vi "Instrucoes.vi"() -> ()   [LabVIEW 2011]
doc: "Esse VI mostra instruções do jogo."
panel:
  in  "OK":bool
  out "Instruções":string
  # "Instruções"
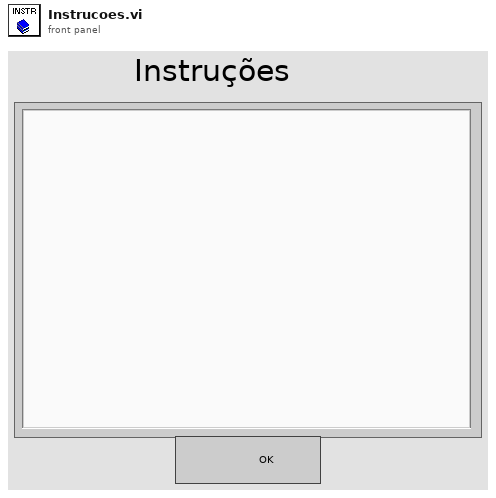
[diagram p1: front panel]
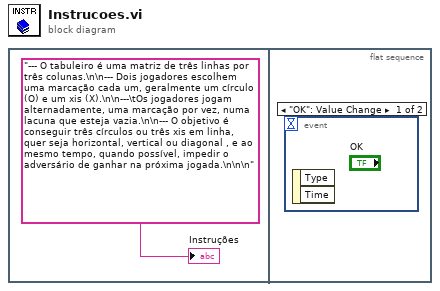
[diagram p0: block diagram]
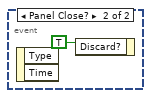
[diagram p2: hidden frame]
diagram:
  n1 = flat-sequence {
    frame #0 {
      "Instruções" <- "--- O tabuleiro é uma matriz de três linhas por três colunas.\n\n--- Dois jogadores escolhem uma marcação cada um, geralmente um círculo (O) e um xis (X).\n\n---\tOs jogadores jogam alternadamente, uma marcação por vez, numa lacuna que esteja vazia.\n\n--- O objetivo é conseguir três círculos ou três xis em linha, quer seja horizontal, vertical ou diagonal , e ao mesmo tempo, quando possível, impedir o adversário de ganhar na próxima jogada.\n\n\n" ("Instruções")
    }
    frame #1 {
      n2 = event shown="[0] \"OK\": Value Change" {
        selector: _ -> [_ _]
        dyn-events: _ -> [_ _]
        timeout: _ -> [_ _]
        event "OK": Value Change {
          n3 = event-data() -> ()  [unwired: 1 in, 2 out]
        }
        event Panel Close? {
          n4 = event-data() -> ()  [unwired: 1 in, 2 out]
          n5 = event-data("Discard?"=TRUE) -> ()  [unwired: 1 in, 1 out]
        }
      }
    }
  }
